vi "Entity Table Info.vi"(8 "error in (no error)":errorcluster, 10 "Entity":refnum<class "Entity.lvclass">, 11 "Database in":refnum<class "Database Platform.lvclass">) -> (0 "error out":errorcluster, 2 "Existing Columns":T1[](array[typedef]), 3 "Database out":refnum<class "Database Platform.lvclass">)   [LabVIEW 2020, in "Conditum.lvlib" / "Database Platform.lvclass"]
uses:
  Database Platform.lvclass
  Entity/Entity.lvclass
  Columns/Type/Type.lvclass
  Column Info.ctl
  Conditum.lvlib
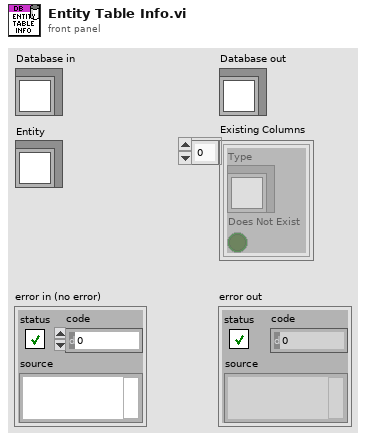
[diagram p1: front panel]
types:
  T1 = typedef "Conditum.lvlib/Column Info.ctl" = cluster{"Type":refnum<class "Type.lvclass">, "Does Not Exist":bool}
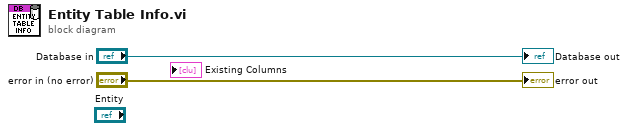
[diagram p0: block diagram]
diagram:
  "error out" <- "error in (no error)"
  "Database out" <- "Database in"
